vi "Format Limit Value.vi"(4 "Value":dbl format="%#_6f") -> (7 "String":string)   [LabVIEW 2020, in "VolatusGUIElements.lvlib" / "BluelinesRedlines.lvclass"]
uses:
  BluelinesRedlines.lvclass
  BluelinesRedlines.lvclass/BluelinesRedlines.ctl
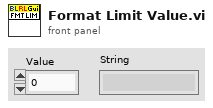
[diagram p1: front panel]
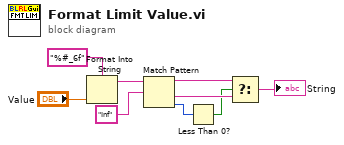
[diagram p0: block diagram]
diagram:
  n1 = Format Into String(format string="%#_6f", "Value") -> (resulting string=w7:string)  [unwired: 2 in, 1 out]
  n2 = Match Pattern(string=w7, regular expression="Inf") -> (before substring=w4:string, after substring=w3:string, offset past match=w5:i32)  [unwired: 1 in, 1 out]
  n3 = Less Than 0?(x=w5) -> (x < 0?=w2:bool)
  n4 = Select(t=w4, s=w2, f=w3) -> (s? t:f=→"String":string)
